vi "SVFA Frequency Response (Real-Im).vi"(0 "stimulus signal X [EUx]":waveform(dbl), 1 "response signal Y [EUy]":waveform(dbl), 2 "window":T8=1 items=["None"=0, "Hanning"=1, "Hamming"=2, "Blackman-Harris"=3, "Exact Blackman"=4, "Blackman"=5, "Flat Top"=6, "4 Term B-Harris "=7, "7 Term B-Harris"=8, "Low Sidelobe"=9, "Force - Exponential"=10, "Blackman Nuttall"=11, "Triangle"=30, "Bartlett-Hanning"=31, "Bohman"=32, "Parzen"=33, "Welch"=34, "Kaiser"=60, "Dolph-Chebyshev"=61, "Gaussian"=62], 5 "error in (no error)":errorcluster, 6 "FRF mode":enum16{"H1", "H2", "H3"}(ring), 7 "averaging parameters":T9={"averaging mode"=enum."No averaging", "weighting mode"=enum."Exponential", "number of averages"=10, "linear mode"=enum."One shot"}, 8 "force/exp settings":T7={"force window [%]"=50.0, "exp window [%]"=10.0} {"exp window [%]" min=0.0 max=100.0 format="%.2f"; "force window [%]" min=0.0 max=100.0 format="%.2f"}, 9 "restart averaging (F)":bool) -> (11 "averaging done":bool, 12 "coherence":cluster{"f0":dbl, "df":dbl, "coherence":dbl[]} {"coherence" format="%.2f"; "df" format="%.2f"; "f0" format="%.2f"}, 13 "averages completed":dbl, 14 "real part [EUy/EUx rms]":cluster{"f0":dbl, "df":dbl, "real part":dbl[]} {"real part" format="%.2f"; "df" format="%.2f"; "f0" format="%.2f"}, 16 "imaginary part [EUy/EUx rms]":T10 {"imaginary part" format="%.2f"; "df" format="%.2f"; "f0" format="%.2f"}, 17 "unit label":string, 18 "spectrum info":T1={"channel name"="", "description"="", "x-axis units"=0, "spectral info"={"spectrum type"=enum."Power [Magnitude^2]", "linear/dB"=enum."linear", "window"=0, "window size"=0, "FFT size"=0}, "engineering units"=0, "custom label"="", "dB reference [EU]"=0.0, "peak units"=enum."rms", "weighting filter"=0, "spectral density?"=FALSE, "unit label"="", "spectrum skewed?"=FALSE, "complimentary spectrum units"=enum."none"} {"x-axis units" items=["Time (s)"=0, "Frequency-CB (Hz)"=1, "Frequency-CPB (Hz)"=1248, "Frequency-Arbitrary (Hz)"=2357, "Quefrency (s)"=2, "Revolutions (rev)"=3, "Order"=4, "Speed (RPM)"=11, "Speed (rad/s)"=21, "Index"=65535]; "weighting filter" items=["Linear", "A-weighting", "B-weighting", "C-weighting", "ITU-R 468-4", "Dolby", "CCITT", "C-message", "Wb", "Wc", "Wd", "We", "Wf", "Wh", "Wj", "Wk", "Wm", "AES17 20 kHz lowpass", "AES17 40 kHz lowpass", "AES17 20 kHz highpass", "AES17 40 kHz highpass"]; "dB reference [EU]" format="%.2f"; "engineering units" items=["custom..."=0, "V"=1, "A"=21, "C"=30, "pC"=31, "s"=32, "-"=29, "Pa"=2, "N"=20, "g"=3, "m/s^2"=4, "m/s"=5, "m"=6, "mm/s"=12, "mm"=13, "micron/s"=14, "micron"=15, "in/s^2"=7, "in/s"=8, "in"=9, "mil/s"=10, "mil"=11, "rad/s^2"=16, "rad/s"=17, "rad"=18, "deg/s^2"=26, "deg/s"=27, "deg"=28, "RPM"=22, "cycle/s^2"=23, "Hz"=24, "cycle"=25, "strain"=19]; "spectral info"."window" items=["None "=0, "Hanning"=1, "Hamming"=2, "Blackman-Harris"=3, "Exact Blackman"=4, "Blackman"=5, "Flat Top"=6, "4 Term B-Harris "=7, "7 Term B-Harris"=8, "Low Sidelobe"=9, "Force - Exponential"=10, "Gaussian"=62]}, 19 "error out":errorcluster)   [LabVIEW 2017]
doc: "Computes the real and imaginary components and coherence of the frequency response of the device under test [DUT]. This VI computes the ratio of the output to the input of the DUT."
uses:
  <vilib>/addons/_NISVFA/_Shared subVIs/Controls/svc_Window [Dual FFT].ctl
  <vilib>/addons/_NISVFA/_Shared subVIs/Controls/svc_Spectrum Info.ctl
  <vilib>/addons/_NISVFA/_Shared subVIs/Controls/svc_X-Axis Units.ctl
  <vilib>/addons/_NISVFA/_Shared subVIs/Controls/svc_Spectrum Type.ctl
  <vilib>/addons/_NISVFA/_Shared subVIs/Controls/svc_Engineering Units Text Ring.ctl
  <vilib>/addons/_NISVFA/_Shared subVIs/Controls/svc_Weighting Filter Text Ring.ctl
  <vilib>/addons/_NISVFA/_Shared subVIs/Controls/svc_Complimentary Spectrum Units.ctl
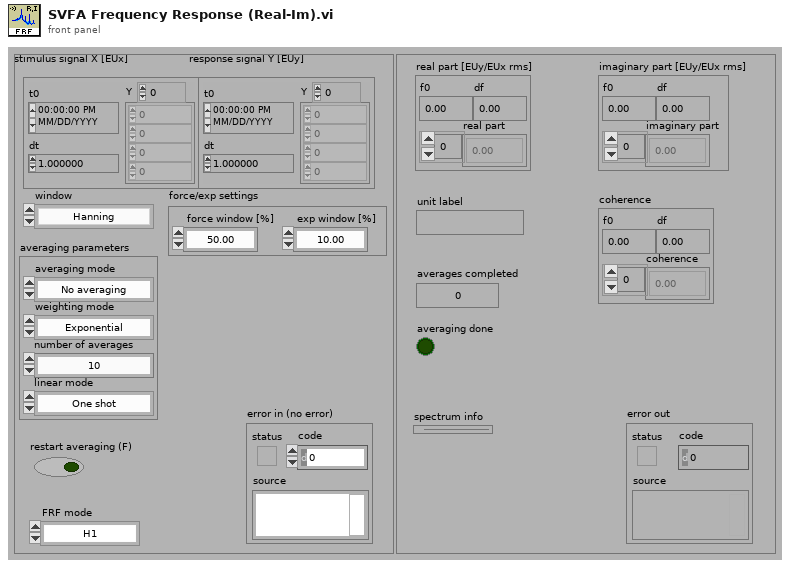
[diagram p1: front panel]
types:
  T1 = typedef "svc_Spectrum Info.ctl" = cluster{"channel name":string, "description":string, "x-axis units":T2, "spectral info":cluster{"spectrum type":T3, "linear/dB":enum16{"linear", "dB"}, "window":u16, "window size":i32, "FFT size":i32}, "engineering units":T4, "custom label":string, "dB reference [EU]":dbl, "peak units":enum16{"rms", "peak", "peak-peak"}, "weighting filter":T5, "spectral density?":bool, "unit label":string, "spectrum skewed?":bool, "complimentary spectrum units":T6}
  T2 = typedef "svc_X-Axis Units.ctl" = u16
  T3 = typedef "svc_Spectrum Type.ctl" = enum16{"FFT Spectrum [complex]", "Amplitude [Magnitude]", "Power [Magnitude^2]", "Cross Spectrum [complex]", "Frequency Response [Complex]"}
  T4 = typedef "svc_Engineering Units Text Ring.ctl" = u16
  T5 = typedef "svc_Weighting Filter Text Ring.ctl" = u16
  T6 = typedef "svc_Complimentary Spectrum Units.ctl" = enum16{"none", "radians", "degrees", "cycles", "imaginary"}
  T7 = cluster{"force window [%]":dbl, "exp window [%]":dbl}
  T8 = typedef "svc_Window [Dual FFT].ctl" = u32
  T9 = cluster{"averaging mode":enum16{"No averaging", "Vector averaging", "RMS averaging", "Peak hold"}, "weighting mode":enum16{"Linear", "Exponential"}, "number of averages":u32, "linear mode":enum16{"One shot", "Auto restart"}}
  T10 = cluster{"f0":dbl, "df":dbl, "imaginary part":dbl[]}
  T11 = enum16{"Cross spectrum", "Frequency response", "Coherent output power"}
  T12 = enum16{"Restart processing", "Continue processing", "Skip processing"}
  T13 = cluster{"f0":dbl, "df":dbl, "complex spectrum":cdb[]}
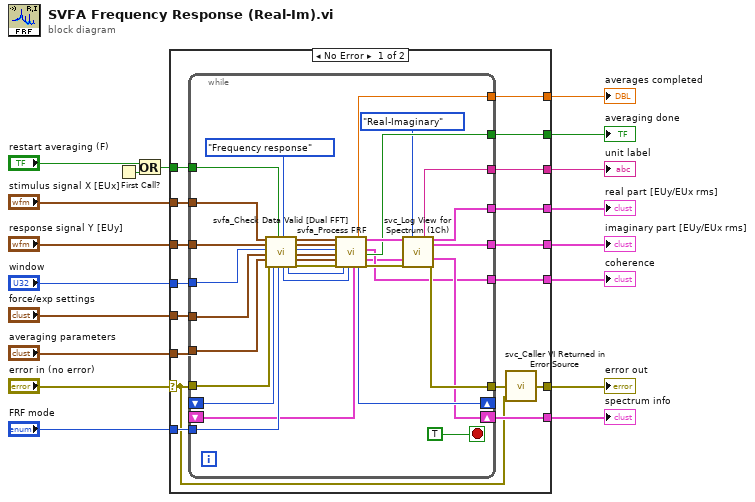
[diagram p0: block diagram]
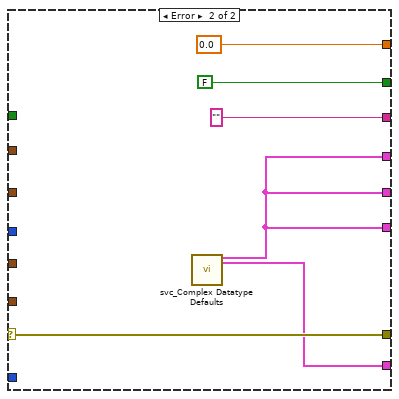
[diagram p2: hidden frame]
diagram:
  n1 = First Call?() -> (First Call?: T/F=w3:bool)
  n2 = Or(x="restart averaging (F)", y=w3) -> (x .or. y?=w1:bool)
  n3 = case shown="No Error" "error in (no error)" {
    selector: "error in (no error)" -> [w19 w74]
    tunnel: "averaging parameters" -> [w30 _]
    tunnel: "window" -> [w32 _]
    tunnel: "force/exp settings" -> [w31 _]
    tunnel: "stimulus signal X [EUx]" -> [w34 _]
    tunnel: "response signal Y [EUy]" -> [w33 _]
    tunnel: [w25 w69] -> w12
    tunnel: [w24 w69] -> w11
    tunnel: [w23 w69] -> w10
    tunnel: [w20 w74] -> w9
    tunnel: [w27 FALSE ("averaging done")] -> w8
    tunnel: [w28 0.0 ("averages completed")] -> w7
    tunnel: w1 -> [w35 _]
    tunnel: "FRF mode" -> [w29 _]
    tunnel: [w26 "" ("unit label (mag or real)")] -> w5
    tunnel: [w22 w70] -> w4
    frame No Error {
      n4 = while {
        tunnel: w34 -> [w43]
        tunnel: w35 -> [w46]
        tunnel: [w48] -> w26
        shift-left: _ -> [w47]
        shift-right: [w51] -> _
        tunnel: w29 -> [w45]
        tunnel: w31 -> [w61]
        tunnel: w30 -> [w59]
        tunnel: w32 -> [w62]
        tunnel: [w39] -> w23
        tunnel: [w63] -> w21
        tunnel: [w38] -> w24
        tunnel: [w64] -> w25
        tunnel: [w66] -> w28
        tunnel: [w50] -> w27
        tunnel: w33 -> [w67]
        tunnel: w19 -> [w68]
        shift-right: [w49] -> w22
        shift-left: _ -> [w37]
        stop <- TRUE stop-if-true
        n5 = call <vilib>:"svfa_Check Data Valid [Dual FFT].vi"("stimulus [X]"=w43, "response [Y]"=w67, "window"=w62, "force/exp settings"=w61, "averaging parameters"=w59, "error in (no error)"=w68, "processing control in"=w47, "restart averaging (F)"=w46, "FRF mode"=w45, "measurement"=T11."Frequency response") -> ("dup FRF mode"=w44:enum16{"H1", "H2", "H3"}, "processing control out"=w52:T12, "dup stimulus [X]"=w58:waveform(dbl), "dup response [Y]"=w57:waveform(dbl), "window"=w56:T8, "dup force/exp settings"=w55:T7, "dup averaging parameters"=w54:T9, "error out"=w53:errorcluster)  [unwired: 2 in]
        n6 = call <vilib>:"svfa_Process FRF.vi"("stimulus signal X [EUx]"=w58, "response signal Y [EUy]"=w57, "window"=w56, "force/exp settings"=w55, "averaging parameters"=w54, "error in (no error)"=w53, "processing control"=w52, "FRF mode"=w44, "spectrum info in"=w37) -> ("averages completed"=w66:dbl, "processing control"=w51:T12, "complex frequency response"=w65:T13, "coherence"=w39:cluster{"f0":dbl, "df":dbl, "coherence":dbl[]}, "averaging done"=w50:bool, "spectrum info out"=w36:T1, "error out"=w40:errorcluster)  [unwired: 2 in, 2 out]
        n7 = call <vilib>:"svc_Log View for Spectrum (1Ch).vi"("complex spectrum"=w65, "View"=enum16{"Mag-Phase", "Real-Imaginary"}."Real-Imaginary", "spectrum info in"=w36, "error in (no error)"=w40) -> ("unit label [mag or real]"=w48:string, "magnitude or real"=w64:cluster{"f0":dbl, "df":dbl, dbl[]}, "phase or imag"=w38:cluster{"f0":dbl, "df":dbl, dbl[]}, "spectrum info out"=w49:T1, "error out"=w63:errorcluster)  [unwired: 6 in, 1 out]
      }
      n8 = call <vilib>:"svc_Caller VI Returned in Error Source.vi"("warning input to caller"=w19, "error in (no error)"=w21) -> ("error out"=w20:errorcluster)  [unwired: 3 in]
    }
    frame Error {
      n9 = call <vilib>:"svc_Complex Datatype Defaults.vi"() -> ("empty spectrum"=w69:cluster{"f0":dbl, "df":dbl, "magnitude":dbl[]}, "dead spectrum info"=w70:T1)  [unwired: 11 in, 7 out]
    }
  }
  "error out" <- w9
  "real part [EUy/EUx rms]" <- w12
  "imaginary part [EUy/EUx rms]" <- w11
  "averaging done" <- w8
  "averages completed" <- w7
  "coherence" <- w10
  "spectrum info" <- w4
  "unit label" <- w5
